vi "sv_Extract Function Info and Unit Info from Spectrum Info.vi"(10 "spectrum info":T2={"channel name"="", "description"="", "x-axis units"=0, "spectral info"={"spectrum type"=enum."Power [Magnitude^2]", "linear/dB"=enum."linear", "window"=0, "window size"=0, "FFT size"=0}, "engineering units"=1, "custom label"="", "dB reference [EU]"=0.0, "peak units"=enum."rms", "weighting filter"=0, "spectral density?"=FALSE, "unit label"="", "spectrum skewed?"=FALSE, "complimentary spectrum units"=enum."none"} {"x-axis units" items=["Time (s)"=0, "Frequency-CB (Hz)"=1, "Frequency-CPB (Hz)"=1248, "Frequency-Arbitrary (Hz)"=2357, "Quefrency (s)"=2, "Revolutions (rev)"=3, "Order"=4, "Speed (RPM)"=11, "Speed (rad/s)"=21, "Index"=65535]; "weighting filter" items=["Linear", "A-weighting", "B-weighting", "C-weighting", "ITU-R 468-4", "Dolby", "CCITT", "C-message", "Wb", "Wc", "Wd", "We", "Wf", "Wh", "Wj", "Wk", "Wm", "AES17 20 kHz lowpass", "AES17 40 kHz lowpass", "AES17 20 kHz highpass", "AES17 40 kHz highpass"]; "dB reference [EU]" format="%.2f"; "engineering units" items=["custom..."=0, "V"=1, "A"=21, "C"=30, "pC"=31, "s"=32, "-"=29, "Pa"=2, "N"=20, "g"=3, "m/s^2"=4, "m/s"=5, "m"=6, "mm/s"=12, "mm"=13, "micron/s"=14, "micron"=15, "in/s^2"=7, "in/s"=8, "in"=9, "mil/s"=10, "mil"=11, "rad/s^2"=16, "rad/s"=17, "rad"=18, "deg/s^2"=26, "deg/s"=27, "deg"=28, "RPM"=22, "cycle/s^2"=23, "Hz"=24, "cycle"=25, "strain"=19]; "spectral info"."window" items=["None "=0, "Hanning"=1, "Hamming"=2, "Blackman-Harris"=3, "Exact Blackman"=4, "Blackman"=5, "Flat Top"=6, "4 Term B-Harris "=7, "7 Term B-Harris"=8, "Low Sidelobe"=9, "Force - Exponential"=10, "Gaussian"=62]}, 11 "spectrum component":T11=33 items=["Magnitude"=32, "Phase"=33, "Real"=34, "Imaginary"=35, "Coherence"=36, "Unknown"=99]) -> (1 "spectrum info.spectrum type string":string, 2 "unit info":T1, 3 "function info":T10 {"function type" items=["Signal"=0, "Speed"=3, "Ratio"=6, "Count"=7, "-"=9, "Level"=10, "-"=19, "Octave Spectrum"=20, "-"=29, "FFT Auto Spectrum"=30, "FFT Cross Spectrum"=40, "Frequency Response"=50, "-"=59, "Event"=90]; "function subtype" items=["Unscaled binary"=0, "Scaled voltage"=1, "Scaled engineering units"=2, "-"=10, "Value"=19, "DC"=11, "AC"=12, "RMS^2"=13, "RMS"=14, "Peak"=15, "Peak to peak"=16, "-"=20, "1/1 octave"=21, "1/3 octave"=22, "1/6 octave"=23, "1/12 octave"=24, "1/24 octave"=25, "-"=30, "Density"=31, "Magnitude"=32, "Phase"=33, "Real"=34, "Imaginary"=35, "Complex"=345, "Coherence"=36, "-"=90, "Unknown"=99]; "X-domain" items=["Time (s)"=0, "Frequency-CB (Hz)"=1, "Frequency-CPB (Hz)"=1248, "Frequency-Arbitrary (Hz)"=2357, "Quefrency (s)"=2, "Revolutions (rev)"=3, "Order"=4, "Speed (RPM)"=11, "Speed (rad/s)"=21, "Index"=65535]})   [LabVIEW 2017]
uses:
  <vilib>/addons/_NISVFA/_Shared subVIs/Controls/NI Spectrum Component.ctl
  <vilib>/addons/_NISVFA/_Shared subVIs/Controls/NI Function Type.ctl
  <vilib>/addons/_NISVFA/_Shared subVIs/Controls/NI Function SubType.ctl
  <vilib>/addons/_NISVFA/_Shared subVIs/Controls/svc_X-Axis Units.ctl
  <vilib>/addons/_NISVFA/_Shared subVIs/Controls/svc_Spectrum Info.ctl
  <vilib>/addons/_NISVFA/_Shared subVIs/Controls/svc_Spectrum Type.ctl
  <vilib>/addons/_NISVFA/_Shared subVIs/Controls/svc_Engineering Units Text Ring.ctl
  <vilib>/addons/_NISVFA/_Shared subVIs/Controls/svc_Weighting Filter Text Ring.ctl
  <vilib>/addons/_NISVFA/_Shared subVIs/Controls/svc_Complimentary Spectrum Units.ctl
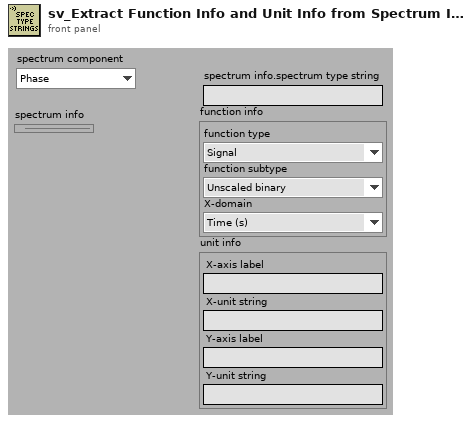
[diagram p1: front panel]
types:
  T1 = cluster{"X-axis label":string, "X-unit string":string, "Y-axis label":string, "Y-unit string":string}
  T2 = typedef "svc_Spectrum Info.ctl" = cluster{"channel name":string, "description":string, "x-axis units":T3, "spectral info":cluster{"spectrum type":T4, "linear/dB":enum16{"linear", "dB"}, "window":u16, "window size":i32, "FFT size":i32}, "engineering units":T5, "custom label":string, "dB reference [EU]":dbl, "peak units":enum16{"rms", "peak", "peak-peak"}, "weighting filter":T6, "spectral density?":bool, "unit label":string, "spectrum skewed?":bool, "complimentary spectrum units":T7}
  T3 = typedef "svc_X-Axis Units.ctl" = u16
  T4 = typedef "svc_Spectrum Type.ctl" = enum16{"FFT Spectrum [complex]", "Amplitude [Magnitude]", "Power [Magnitude^2]", "Cross Spectrum [complex]", "Frequency Response [Complex]"}
  T5 = typedef "svc_Engineering Units Text Ring.ctl" = u16
  T6 = typedef "svc_Weighting Filter Text Ring.ctl" = u16
  T7 = typedef "svc_Complimentary Spectrum Units.ctl" = enum16{"none", "radians", "degrees", "cycles", "imaginary"}
  T8 = typedef "NI Function Type.ctl" = u16
  T9 = typedef "NI Function SubType.ctl" = u16
  T10 = cluster{"function type":T8, "function subtype":T9, "X-domain":T3}
  T11 = typedef "NI Spectrum Component.ctl" = u16
  T12 = cluster{"function type":T8, "function subtype":T9, "X-Dimension":T3}
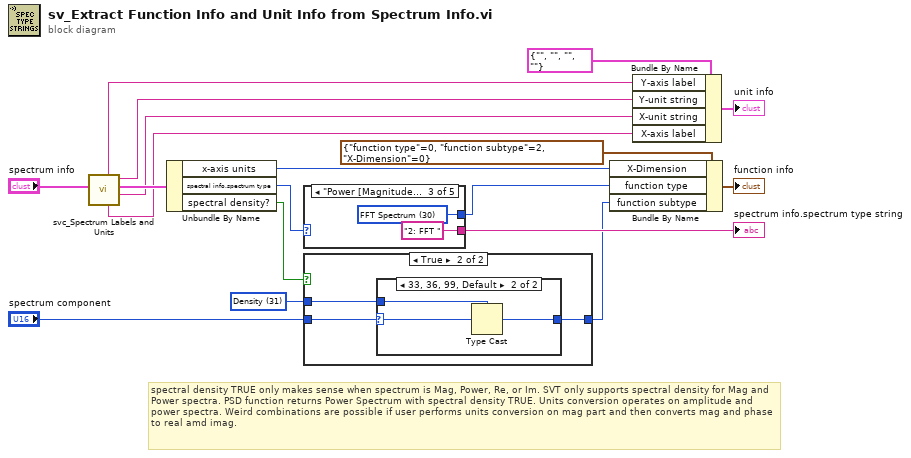
[diagram p0: block diagram]
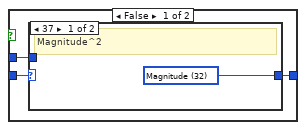
[diagram p2: hidden frame]
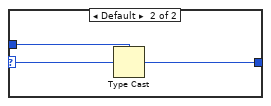
[diagram p3: hidden frame]
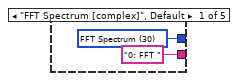
[diagram p5: hidden frame]
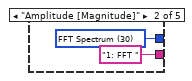
[diagram p6: hidden frame]
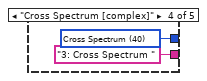
[diagram p7: hidden frame]
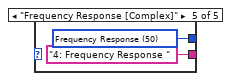
[diagram p8: hidden frame]
diagram:
  w1 = T9 31 items=["Unscaled binary"=0, "Scaled voltage"=1, "Scaled engineering units"=2, "-"=10, "Value"=19, "DC"=11, "AC"=12, "RMS^2"=13, "RMS"=14, "Peak"=15, "Peak to peak"=16, "-"=20, "1/1 octave"=21, "1/3 octave"=22, "1/6 octave"=23, "1/12 octave"=24, "1/24 octave"=25, "-"=30, "Density"=31, "Magnitude"=32, "Phase"=33, "Real"=34, "Imaginary"=35, "Complex"=345, "Coherence"=36, "-"=90, "Unknown"=99] ("function subtype")
  # "spectral density TRUE only makes sense when spectrum is Mag, Power, Re, or Im. SVT only supports spectral density for Mag and Power spectra. PSD function returns Power Spectrum with spectral density TRUE. Units conversion operates on amplitude and power spectra. Weird combinations are possible if user performs units conversion on mag part and then converts mag and phase to real amd imag."
  n1 = call <vilib>:"svc_Spectrum Labels and Units.vi"("spectrum info in"="spectrum info") -> ("x-axis unit label"=w5:string, "spectrum info out"=w8:T2, "unit label"=w4:string, "x-axis label"=w6:string, "y-axis label"=w3:string)  [unwired: 5 in, 1 out]
  n2 = Unbundle By Name(w8) -> ("x-axis units"=w10:T3, "spectral info.spectrum type"=w12:T4, "spectral density?"=w11:bool)
  n3 = case shown="\"Power [Magnitude^2]\"" w12 {
    tunnel: ["0: FFT " ("t") "1: FFT " ("t") "2: FFT " ("t") "3: Cross Spectrum " ("t") "4: Frequency Response " ("t")] -> w17
    tunnel: [w19 w21 w23 w25 w27] -> w13
    frame "FFT Spectrum [complex]", Default {
      w19 = T8 30 items=["Signal"=0, "Level"=10, "Octave Spectrum"=20, "FFT Spectrum"=30, "Cross Spectrum"=40, "Frequency Response"=50, "Ratio"=6, "Count"=7] ("function type")
    }
    frame "Amplitude [Magnitude]" {
      w21 = T8 30 items=["Signal"=0, "Level"=10, "Octave Spectrum"=20, "FFT Spectrum"=30, "Cross Spectrum"=40, "Frequency Response"=50, "Ratio"=6, "Count"=7] ("function type")
    }
    frame "Power [Magnitude^2]" {
      w23 = T8 30 items=["Signal"=0, "Level"=10, "Octave Spectrum"=20, "FFT Spectrum"=30, "Cross Spectrum"=40, "Frequency Response"=50, "Ratio"=6, "Count"=7] ("function type")
    }
    frame "Cross Spectrum [complex]" {
      w25 = T8 40 items=["Signal"=0, "Level"=10, "Octave Spectrum"=20, "FFT Spectrum"=30, "Cross Spectrum"=40, "Frequency Response"=50, "Ratio"=6, "Count"=7] ("function type")
    }
    frame "Frequency Response [Complex]" {
      w27 = T8 50 items=["Signal"=0, "Level"=10, "Octave Spectrum"=20, "FFT Spectrum"=30, "Cross Spectrum"=40, "Frequency Response"=50, "Ratio"=6, "Count"=7] ("function type")
    }
  }
  "spectrum info.spectrum type string" <- w17
  n4 = case shown="True" w11 {
    tunnel: "spectrum component" -> [w31 w38]
    tunnel: [w30 w37] -> w15
    tunnel: w1 -> [w29 w36]
    frame False {
      n5 = case shown="37" w31 {
        selector: w31 -> [_ w34]
        tunnel: [w32 w33] -> w30
        tunnel: w29 -> [_ w35]
        frame 37 {
          w32 = T9 32 items=["Unscaled binary"=0, "Scaled voltage"=1, "Scaled engineering units"=2, "-"=10, "Value"=19, "DC"=11, "AC"=12, "RMS^2"=13, "RMS"=14, "Peak"=15, "Peak to peak"=16, "-"=20, "1/1 octave"=21, "1/3 octave"=22, "1/6 octave"=23, "1/12 octave"=24, "1/24 octave"=25, "-"=30, "Density"=31, "Magnitude"=32, "Phase"=33, "Real"=34, "Imaginary"=35, "Complex"=345, "Coherence"=36, "-"=90, "Unknown"=99] ("function subtype")
          # "Magnitude^2"
        }
        frame Default {
          n6 = Type Cast(type=w35, x=w34) -> (*(type *) &x=w33:T9)
        }
      }
    }
    frame True {
      n7 = case shown="33, 36, 99, Default" w38 {
        selector: w38 -> [_ w42]
        tunnel: [w39 w40] -> w37
        tunnel: w36 -> [w39 w41]
        frame 32, 34, 35, 37, 345 {
        }
        frame 33, 36, 99, Default {
          n8 = Type Cast(type=w41, x=w42) -> (*(type *) &x=w40:T9)
        }
      }
    }
  }
  n9 = Bundle By Name(cluster=T12 {"function type"=0, "function subtype"=2, "X-Dimension"=0} ("function info"), "X-Dimension"=w10, "function type"=w13, "function subtype"=w15) -> (→"function info":T12)
  n10 = Bundle By Name(cluster=T1 {"X-axis label"="", "X-unit string"="", "Y-axis label"="", "Y-unit string"=""} ("unit info"), "Y-axis label"=w3, "Y-unit string"=w4, "X-unit string"=w5, "X-axis label"=w6) -> (→"unit info":T1)
